vi "ScanDeviceReadCharacteristicUUID.vi"() -> (2 "Table Control":string[][](table))   [LabVIEW 2019]
uses:
  C:/Users/chrismadlax/Desktop/LabVIEW-BLE-Driver/BLELib.dll
  BLELib.dll
panel:
  in  "ReadC_UUID":bool
  in  "ScanDevice":bool
  out "INIT":bool
  in  "Listbox":i32(listbox)
  out "Retry":i32
  out "Scanning":string
  out "Pair Result":string
  # "A4:DA:32:0D:F5:E2"
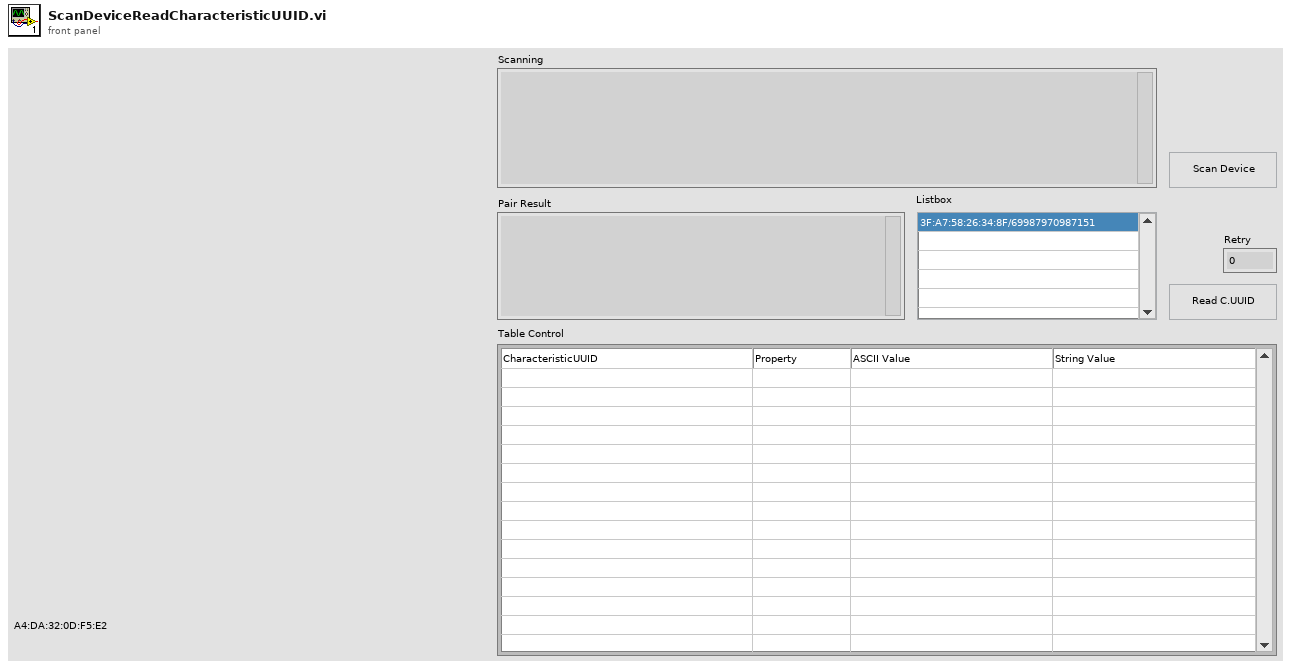
[diagram p1: front panel]
types:
  T1 = cluster{"BLElib":refnum<k24>, "RawAddress":u64[]}
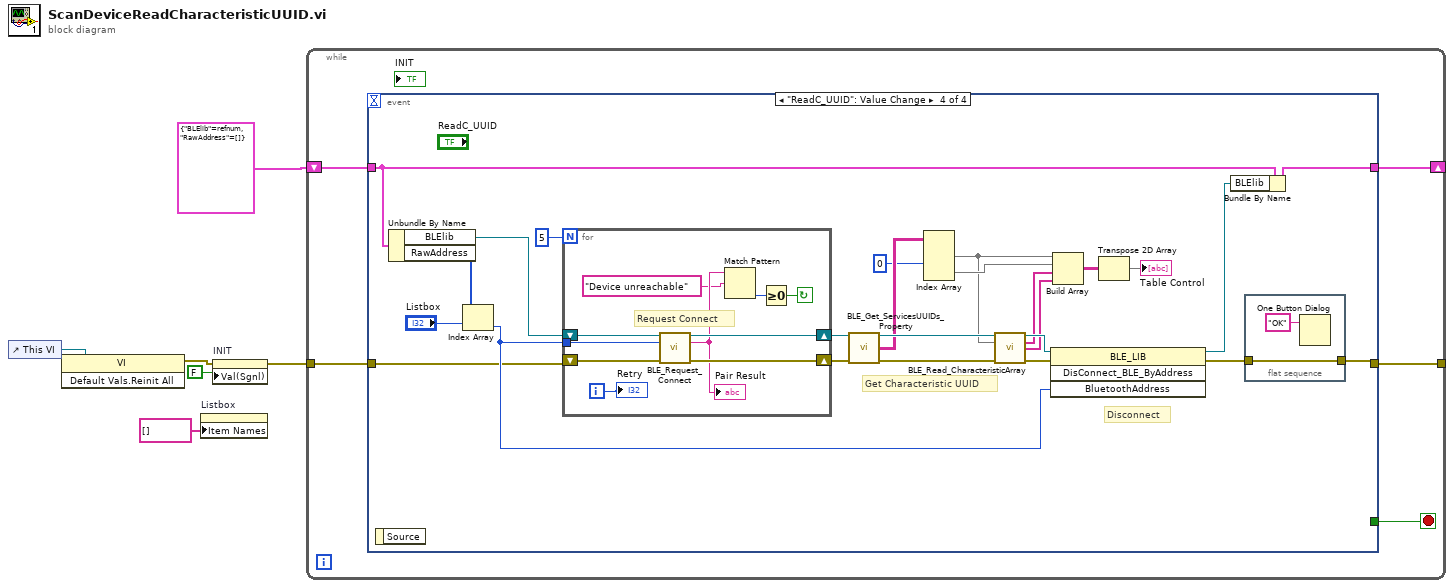
[diagram p0: block diagram]
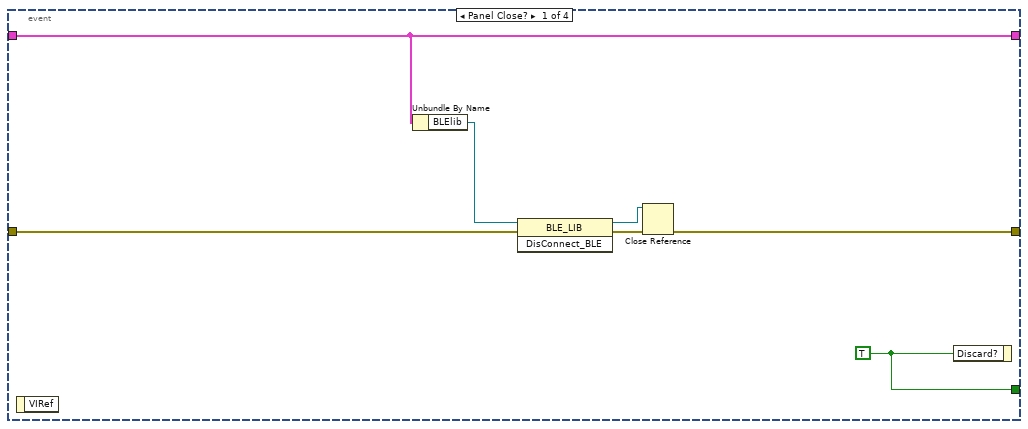
[diagram p2: hidden frame]
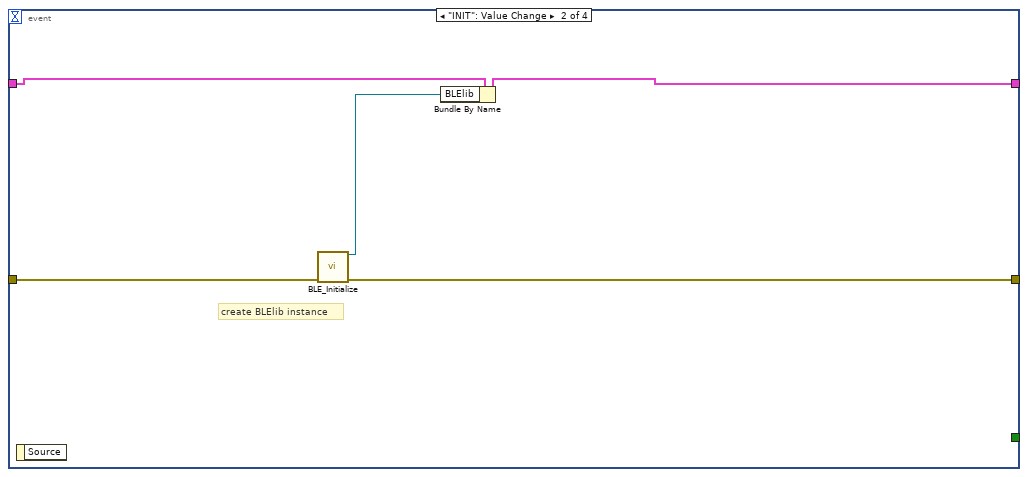
[diagram p3: hidden frame]
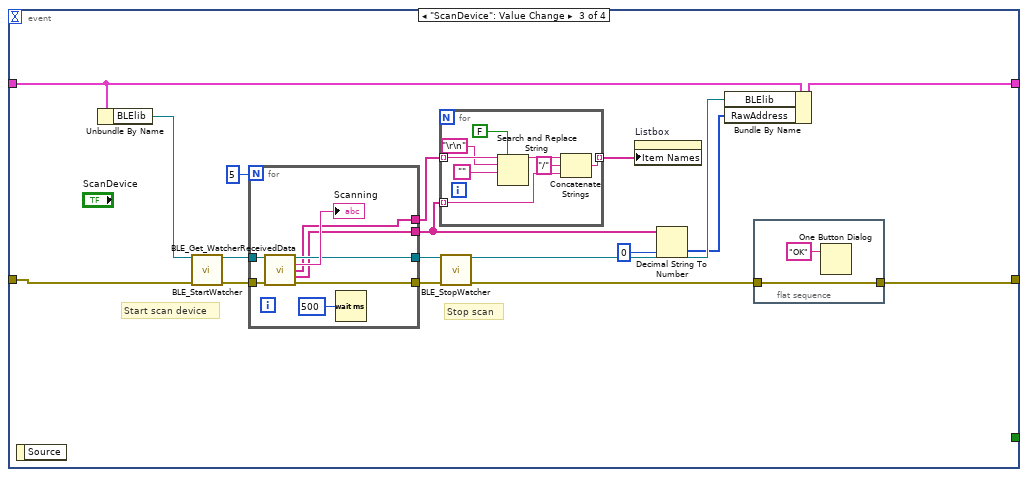
[diagram p4: hidden frame]
diagram:
  n1 = control-ref of="This VI"() -> (w3:refnum<vi>)
  n2 = invoke class="VI" method="Default Vals.Reinit All"(reference=w3) -> (error out=w2:errorcluster)  [unwired: 2 in, 2 out]
  n3 = property on="Listbox" class="LstBox (strict)"("Item Names"=string[] []) -> ()  [unwired: 2 in, 2 out]
  n4 = property on="INIT" class="Bool (strict)"(error in=w2, "Val(Sgnl)"=FALSE ("Value (Signaling)")) -> (error out=w6:errorcluster)  [unwired: 1 in, 1 out]
  n5 = while {
    shift-right: [w8] -> _
    shift-left: T1 {"BLElib"=refnum, "RawAddress"=[]} -> [w7]
    tunnel: w6 -> [w10]
    tunnel: [w9] -> _
    stop <- w11 stop-if-true
    n6 = event shown="[3] \"ReadC_UUID\": Value Change" {
      selector: _ -> [_ _ _ _]
      dyn-events: _ -> [_ _ _ _]
      timeout: _ -> [_ _ _ _]
      tunnel: [w18 _ _ _] -> w11
      tunnel: w10 -> [w15 w23 w34 w66]
      tunnel: [w14 w22 w26 w59] -> w9
      tunnel: [w13 w20 w32 w61] -> w8
      tunnel: w7 -> [w13 w21 w31 w62]
      event Panel Close? {
        w18 = TRUE ("Discard?")
        n7 = event-data() -> ()  [unwired: 1 in, 1 out]
        n8 = Unbundle By Name(w13) -> ("BLElib"=w12:refnum<k24>)
        n9 = invoke class="BLE_LIB" method="DisConnect_BLE"(reference=w12, error in=w15) -> (reference out=w17:refnum<k24>, error out=w16:errorcluster)  [unwired: 1 in, 1 out]
        n10 = Close Reference(reference=w17, error in (no error)=w16) -> (error out=w14:errorcluster)
        n11 = event-data("Discard?"=w18) -> ()  [unwired: 1 in, 1 out]
      }
      event "INIT": Value Change {
        # "create BLElib instance"
        n12 = event-data() -> ()  [unwired: 1 in, 1 out]
        n13 = call "BLE_Initialize.vi"("error in (no error)"=w23) -> (".NET Refnum out"=w19:refnum<k24>, "error out"=w22:errorcluster)  [unwired: 13 in]
        n14 = Bundle By Name(cluster=w21, "BLElib"=w19) -> (w20:T1)
      }
      event "ScanDevice": Value Change {
        # "Stop scan"
        # "Start scan device"
        n15 = event-data() -> ()  [unwired: 1 in, 1 out]
        n16 = Unbundle By Name(w31) -> ("BLElib"=w30:refnum<k24>)
        n17 = call "BLE_StartWatcher.vi"(".NET Refnum in"=w30, "error in (no error)"=w34) -> (".NET Refnum out"=w37:refnum<k24>, "error out"=w36:errorcluster)  [unwired: 11 in, 1 out]
        n18 = for {
          N: 5 -> [_]
          tunnel: [w53] -> w38
          tunnel: w37 -> [w57]
          tunnel: [w54] -> w39
          tunnel: w36 -> [w55]
          tunnel: [w52] -> w40
          tunnel: [w51] -> w24
          n19 = call "BLE_Get_WatcherReceivedData.vi"(".NET Refnum in"=w57, "error in (no error)"=w55) -> (".NET Refnum out"=w53:refnum<k24>, "Watcher Response"=→"Scanning":string, "Bluetooth Addr"=w52:string[], "Bluetooth Raw Addr"=w51:string[], "error out"=w54:errorcluster)  [unwired: 6 in, 3 out]
          n20 = Wait (ms)(milliseconds to wait=u32 500) -> ()  [unwired: 1 out]
        }
        n21 = for {
          tunnel: w40 -> [w50] mode=indexing
          tunnel: [w45] -> w27 mode=indexing
          tunnel: w24 -> [w44] mode=indexing
          n22 = Search and Replace String(replace all?=FALSE ("replace all? (F)"), input string=w50, search string="\r\n", replace string="") -> (result string=w49:string)  [unwired: 4 in, 3 out]
          n23 = Concatenate Strings(w49, "/" ("string"), w44) -> (w45:string)
        }
        n24 = call "BLE_StopWatcher.vi"(".NET Refnum in"=w38, "error in (no error)"=w39) -> (".NET Refnum out"=w29:refnum<k24>, "error out"=w33:errorcluster)  [unwired: 11 in, 1 out]
        n25 = property on="Listbox" class="LstBox (strict)"("Item Names"=w27) -> ()  [unwired: 2 in, 2 out]
        n26 = Decimal String To Number(string=w24, default (0L)=u64 0 ("default (0 I32)")) -> (number=w28:u64[])  [unwired: 1 in, 1 out]
        n27 = Bundle By Name(cluster=w31, "BLElib"=w29, "RawAddress"=w28) -> (w32:T1)
        n28 = flat-sequence {
          tunnel: w33 -> [w42]
          tunnel: [w42] -> w26
          frame #0 {
            n29 = One Button Dialog(message="OK") -> ()  [unwired: 1 in, 1 out]
          }
        }
      }
      event "ReadC_UUID": Value Change {
        # "Disconnect"
        # "Get Characteristic UUID"
        n30 = event-data() -> ()  [unwired: 1 in, 1 out]
        n31 = Unbundle By Name(w62) -> ("BLElib"=w63:refnum<k24>, "RawAddress"=w64:u64[])
        n32 = Index Array(array=w64, index="Listbox") -> (element=w83:u64)
        n33 = for {
          N: 5 -> [_]
          tunnel: w83 -> [w93]
          shift-right: [w91] -> w70
          shift-left: w66 -> [w95]
          shift-right: [w92] -> w69
          shift-left: w63 -> [w94]
          i -> [w86]
          stop <- w87 continue-if-true
          # "Request Connect"
          n34 = call "BLE_Request_Connect.vi"(".NET Refnum in"=w94, "BluetoothAddress"=w93, "error in (no error)"=w95) -> (".NET Refnum out"=w92:refnum<k24>, "ConnectBLE"=w90:string, "error out"=w91:errorcluster)  [unwired: 10 in]
          "Pair Result" <- w90
          n35 = Match Pattern(string=w90, regular expression="Device unreachable") -> (offset past match=w88:i32)  [unwired: 1 in, 3 out]
          n36 = Greater Or Equal To 0?(x=w88) -> (x >= 0?=w87:bool)
          "Retry" <- w86
        }
        n37 = call "BLE_Get_ServicesUUIDs_Property.vi"(".NET Refnum in"=w69, "error in (no error)"=w70) -> (".NET Refnum out"=w79:refnum<k24>, "Char Val-Property"=w77:string[][], "error out"=w78:errorcluster)  [unwired: 11 in]
        n38 = Index Array(array=w77, index (col) #1=0 ("disabled index (col)")) -> (element #1=w74:string[], element #2=w75:string[])  [unwired: 3 in]
        n39 = call "BLE_Read_CharacteristicArray.vi"(".NET Refnum in"=w79, "ServicesUUIDs Extract Value"=w74, "error in (no error)"=w78) -> (".NET Refnum out"=w80:refnum<k24>, "ServicesUUIDs ASCII Value"=w71:string[], "ServicesUUIDs Value"=w72:string[], "error out"=w81:errorcluster)  [unwired: 9 in]
        n40 = invoke class="BLE_LIB" method="DisConnect_BLE_ByAddress"(reference=w80, error in=w81, "BluetoothAddress"=w83) -> (reference out=w60:refnum<k24>, error out=w65:errorcluster)  [unwired: 1 in, 2 out]
        n41 = Build Array(w74, w75, w71, w72) -> (w73:string[][])
        n42 = Transpose 2D Array(2D array=w73) -> (transposed array=→"Table Control":string[][])
        n43 = Bundle By Name(cluster=w62, "BLElib"=w60) -> (w61:T1)
        n44 = flat-sequence {
          tunnel: w65 -> [w85]
          tunnel: [w85] -> w59
          frame #0 {
            n45 = One Button Dialog(message="OK") -> ()  [unwired: 1 in, 1 out]
          }
        }
      }
    }
  }
